vi "SGL to U16.vi"(11 "SGL":sgl) -> (3 "U16":u16[](array[numeric]))   [LabVIEW 2019, in "Modbus DataType Conversation.lvlib"]
uses:
  Modbus DataType Conversation.lvlib
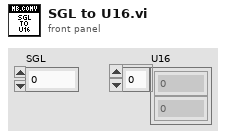
[diagram p1: front panel]
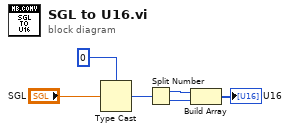
[diagram p0: block diagram]
diagram:
  n1 = Type Cast(type=u32 0, x="SGL") -> (*(type *) &x=w6:u32)
  n2 = Split Number(x=w6) -> (hi(x)=w3:u16, lo(x)=w2:u16)
  n3 = Build Array(w3, w2) -> (→"U16":u16[])
